vi "Enc to XY.vi"(8 "Factor":cluster{"Kx":dbl, "Ky":dbl, "Kz":dbl}={"Kx"=0.02114, "Ky"=0.0245, "Kz"=0.0705} {"Kz" format="%#_13g"; "Ky" format="%#_13g"; "Kx" format="%#_13g"}, 10 "Encoders":T1) -> (0 "Z":dbl, 2 "Distance":cluster{"X":dbl, "Y":dbl})   [LabVIEW 2020]
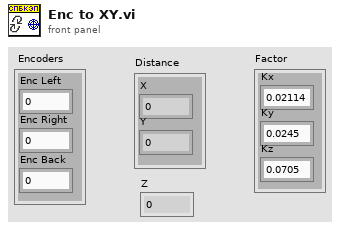
[diagram p1: front panel]
types:
  T1 = cluster{"Enc Left":dbl, "Enc Right":dbl, "Enc Back":dbl}
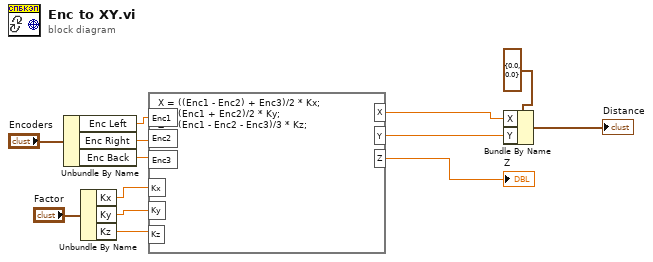
[diagram p0: block diagram]
diagram:
  n1 = Unbundle By Name("Encoders") -> ("Enc Left"=w8:dbl, "Enc Right"=w7:dbl, "Enc Back"=w6:dbl)
  n2 = Unbundle By Name("Factor") -> ("Kx"=w10:dbl, "Ky"=w11:dbl, "Kz"=w12:dbl)
  n3 = formula code="X = ((Enc1 - Enc2) + Enc3)/2 * Kx;\nY = (Enc1 + Enc2)/2 * Ky;\nZ = (Enc1 - Enc2 - Enc3)/3 * Kz;"("Enc1"=w8, "Enc2"=w7, "Enc3"=w6, "Ky"=w11, "Kx"=w10, "Kz"=w12) -> ("X"=w5:dbl, "Y"=w1:dbl, "Z"=→"Z":dbl)
  n4 = Bundle By Name(cluster=cluster{"X":dbl, "Y":dbl} {"X"=0.0, "Y"=0.0} ("Distance"), "X"=w5, "Y"=w1) -> (→"Distance":cluster{"X":dbl, "Y":dbl})
